vi "uTransport_SendMsg Core.vi"(8 "error in (no error)":errorcluster, 10 "Msg":refnum<class "uMsg.lvclass">, 11 "uActor in":refnum<class "uActor.lvclass">) -> (0 "error out":errorcluster, 3 "uActor out":refnum<class "uActor.lvclass">)   [LabVIEW 2021, in "uFramework.lvlib" / "uActor.lvclass"]
uses:
  uActor.lvclass
  uMsg/uMsg.lvclass
  uActor.lvclass/uActor.ctl
  uMsg/uMsg.lvclass/uMsg.ctl
  uTransport_uActor/uTransport_uActor.lvclass/uTransport_uActor.ctl
  uTransport_uActor/uTransport_uActor_SendMsg.vi
  uMsg/uMsg Update Timestamp.vi
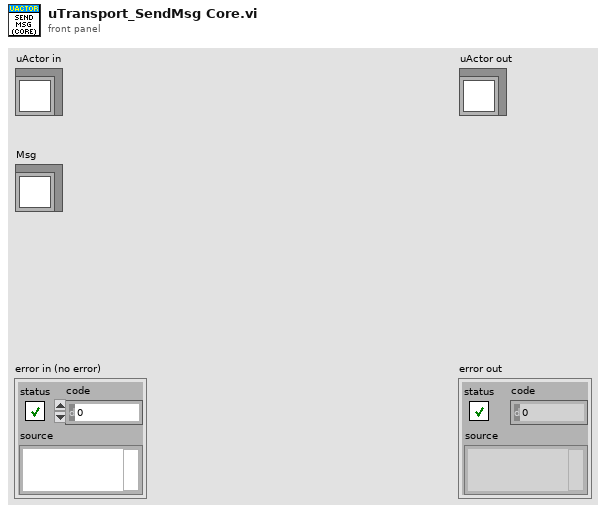
[diagram p1: front panel]
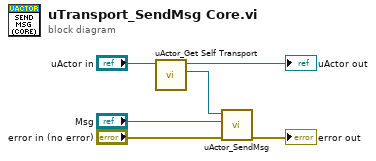
[diagram p0: block diagram]
diagram:
  n1 = call "uActor_Get Self Transport.vi"("uActor in"="uActor in") -> ("Actor Transport"=w4:refnum<class "uTransport_uActor.lvclass">, "uActor out"=→"uActor out":refnum<class "uActor.lvclass">)  [unwired: 9 in]
  n2 = call "uActor_SendMsg.vi"("error in (no error)"="error in (no error)", "Msg"="Msg", "uActor Transport"=w4) -> ("error out"=→"error out":errorcluster)  [unwired: 8 in]
